vi "Read (Limit).vi"(8 "error in (no error)":errorcluster, 11 "VISA resource name":refnum<visa-resource-name>) -> (0 "error out":errorcluster, 1 "Upper Limit Failure Count":dbl, 2 "Lower Limit Failure Count":dbl, 3 "VISA resource name out":refnum<visa-resource-name>, 4 "Total  Failure Count":dbl, 5 "Limit Status":bool, 6 "Total  Pass Count":dbl)   [LabVIEW 2013, in "Counter.lvlib" / "PICOTEST U62XXA series.lvlib"]
doc: "Reads and returns the most recent results of the Limit test.\n\n<B>Note:</B>\n\nIf no valid result exists, 0 is returned."
uses:
  PICOTEST U62XXA series.lvlib
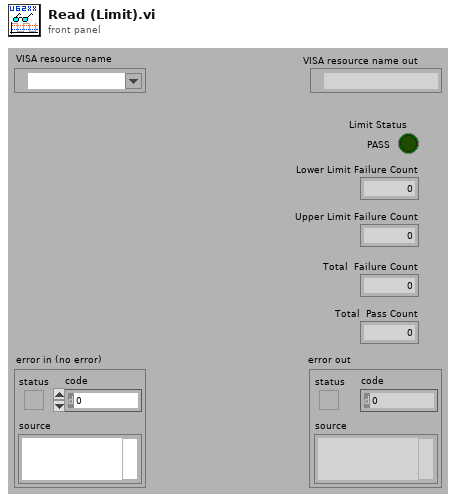
[diagram p1: front panel]
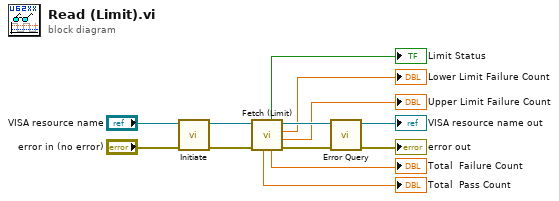
[diagram p0: block diagram]
diagram:
  n1 = call "Initiate.vi"("error in (no error)"="error in (no error)", "VISA resource name"="VISA resource name") -> ("error out"=w6:errorcluster, "VISA resource name out"=w8:refnum<visa-resource-name>)  [unwired: 8 in]
  n2 = call "Fetch (Limit).vi"("error in (no error)"=w6, "VISA resource name"=w8) -> ("error out"=w11:errorcluster, "Upper Limit Failure Count"=→"Upper Limit Failure Count":dbl, "Lower Limit Failure Count"=→"Lower Limit Failure Count":dbl, "VISA resource name out"=w13:refnum<visa-resource-name>, "Total  Failure Count"=→"Total  Failure Count":dbl, "Limit Status"=→"Limit Status":bool, "Total  Pass Count"=→"Total  Pass Count":dbl)  [unwired: 3 in]
  n3 = call "Error Query.vi"("error in (no error)"=w11, "VISA resource name"=w13) -> ("error out"=→"error out":errorcluster, "VISA resource name out"=→"VISA resource name out":refnum<visa-resource-name>)  [unwired: 6 in, 2 out]
